vi "SiosIfmEnvSensorCount.vi"(1 "Device Number":i32) -> (0 "Sensor Count":u32)   [LabVIEW 2009]
uses:
  siosifm.dll
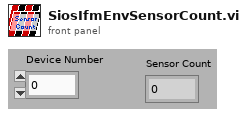
[diagram p1: front panel]
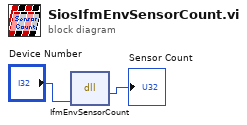
[diagram p0: block diagram]
diagram:
  n1 = dll-call lib="C:/WORK/Artem/RE-10/SIOS_IfmDLL/siosifm.dll" fn="IfmEnvSensorCount"("devNumber"="Device Number") -> ("sensor_count"=→"Sensor Count":u32)  [unwired: 4 in, 2 out]
